vi "TCP Send Response.vi"(8 "error in (no error)":errorcluster, 10 "JSON Response String":string, 11 "TCP Network Connection in":refnum<k5>) -> (0 "error out":errorcluster)   [LabVIEW 2015]
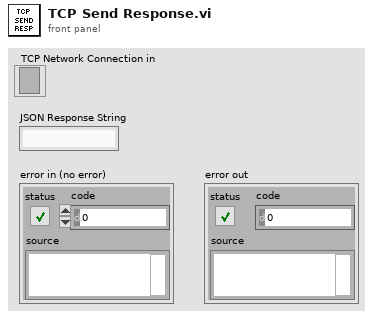
[diagram p1: front panel]
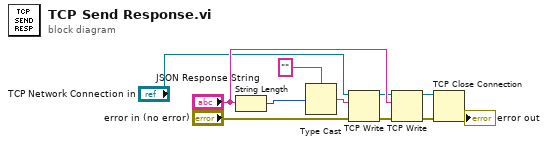
[diagram p0: block diagram]
diagram:
  n1 = String Length(string="JSON Response String") -> (length=w3:i32)
  n2 = Type Cast(type="" ("format string"), x=w3) -> (*(type *) &x=w6:string)
  n3 = TCP Write(connection ID="TCP Network Connection in", data in=w6, error in (no error)="error in (no error)") -> (connection ID out=w5:refnum<k5>, error out=w7:errorcluster)  [unwired: 1 in, 1 out]
  n4 = TCP Write(connection ID=w5, data in="JSON Response String", error in (no error)=w7) -> (connection ID out=w9:refnum<k5>, error out=w10:errorcluster)  [unwired: 1 in, 1 out]
  n5 = TCP Close Connection(connection ID=w9, error in (no error)=w10) -> (error out=→"error out":errorcluster)  [unwired: 1 in, 1 out]
